vi "SERVO.vi"(3 "freq [Hz]":dbl=50.0, 4 "null offset":bool, 5 "position [%FS]":dbl(slide) scale=-200.0..200.0) -> (0 "duty cycle [%]":dbl, 1 "pulse width [ms]":dbl=1.5, 2 "offset [%FS]":dbl)   [LabVIEW 2014]
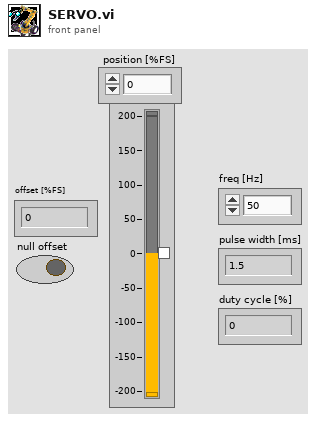
[diagram p1: front panel]
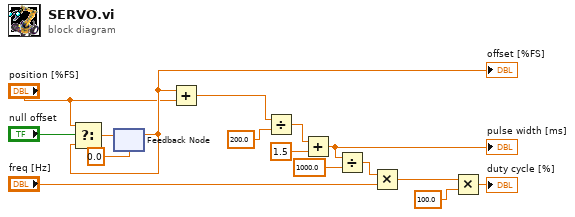
[diagram p0: block diagram]
diagram:
  n1 = feedback #1(0.0 ("position [%FS]")) -> (w7:dbl)
  "offset [%FS]" <- w7
  n2 = Select(t="position [%FS]", s="null offset", f=w7) -> (s? t:f=w9:dbl)
  n3 = feedback-in #1(w9) -> ()
  n4 = Add(x=w7, y="position [%FS]") -> (x+y=w8:dbl)
  n5 = Divide(x=w8, y=200.0) -> (x/y=w15:dbl)
  n6 = Add(x=w15, y=1.5) -> (x+y=w13:dbl)
  "pulse width [ms]" <- w13
  n7 = Divide(x=w13, y=1000.0) -> (x/y=w5:dbl)
  n8 = Multiply(x=w5, y="freq [Hz]") -> (x*y=w2:dbl)
  n9 = Multiply(x=w2, y=100.0) -> (x*y=→"duty cycle [%]":dbl)
